vi "DIM_Read Item (Sourcer, SysLab).vi"(8 "error in (no error)":errorcluster, 9 "SysLabel":string, 10 "Sourcer":string, 11 "UI_Actor in":refnum<class "UI_Actor.lvclass">) -> (0 "error out":errorcluster, 1 "Found?":bool, 2 "DIM Item":T1, 3 "UI_Actor out":refnum<class "UI_Actor.lvclass">)   [LabVIEW 2020, in "UI_Actor.lvlib" / "UI_Actor.lvclass"]
uses:
  UI_Actor.lvclass
  support/Databox.lvlibp/TypesTools/Config/Config.lvclass
  support/Databox.lvlibp/TypesTools/Data/Data.lvclass
  ctl_InternalMapItem.ctl
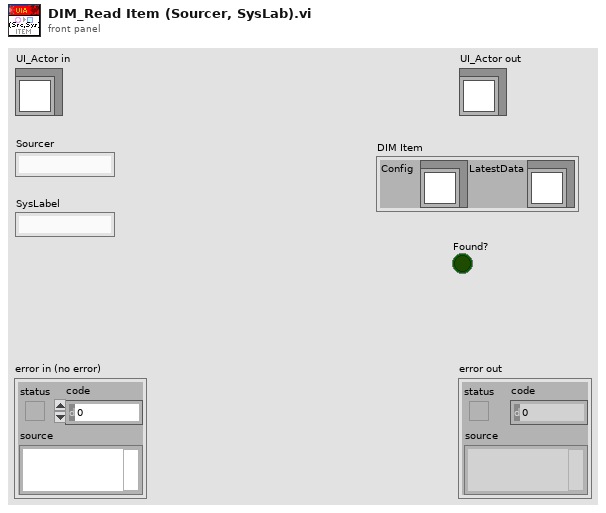
[diagram p1: front panel]
types:
  T1 = typedef "UI_Actor.lvlib/UI_Actor.lvclass/ctl_InternalMapItem.ctl" = cluster{"Config":refnum<class "Config.lvclass">, "LatestData":refnum<class "Data.lvclass">}
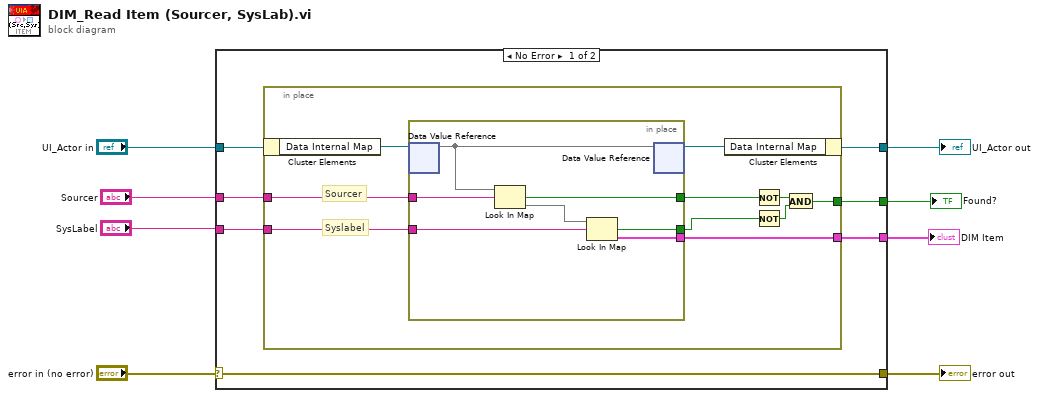
[diagram p0: block diagram]
diagram:
  n1 = case shown="No Error" "error in (no error)" {
    selector: "error in (no error)" -> [w15 w34]
    tunnel: [w15 w34] -> w7
    tunnel: [w13 w33] -> w5
    tunnel: "UI_Actor in" -> [w14 w33]
    tunnel: "Sourcer" -> [w12 _]
    tunnel: [w11 _] -> w4
    tunnel: [w10 _] -> w3
    tunnel: "SysLabel" -> [w9 _]
    frame No Error {
      n2 = in-place {
        in-place-border: w12 -> [w23]
        in-place-border: [w22] -> w11
        in-place-border: [w16] -> w10
        in-place-border: w9 -> [w20]
        # "Syslabel"
        # "Sourcer"
        n3 = in-place-cluster #1(w14) -> ("Data Internal Map"=w25:refnum<data-value>)
        n4 = in-place {
          in-place-border: w23 -> [w31]
          in-place-border: [w27] -> w22
          in-place-border: [w30] -> w21
          in-place-border: w20 -> [w28]
          in-place-border: [w26] -> w19
          n5 = in-place-dvr #2(w25) -> (w32:map{string, map{string, T1}})  [unwired: 1 out]
          n6 = Look In Map(map=w32, key=w31) -> (key not found?=w30:bool, value=w29:map{string, T1})  [unwired: 1 in]
          n7 = Look In Map(map=w29, key=w28) -> (key not found?=w26:bool, value=w27:T1)  [unwired: 1 in]
          n8 = in-place-dvr #2(w32) -> (w24:refnum<data-value>)  [unwired: 1 out]
        }
        n9 = in-place-cluster #1("Data Internal Map"=w24) -> (w13:refnum<class "UI_Actor.lvclass">)
        n10 = Not(x=w21) -> (.not. x?=w18:bool)
        n11 = Not(x=w19) -> (.not. x?=w17:bool)
        n12 = And(x=w18, y=w17) -> (x .and. y?=w16:bool)
      }
    }
    frame Error {
    }
  }
  "error out" <- w7
  "UI_Actor out" <- w5
  "DIM Item" <- w4
  "Found?" <- w3
